vi "Z900_navX_Internal_SendIntegrationControl.vi"(8 "error in (no error)":errorcluster, 9 "Integration Control Register":T7 items=["UNDEFINED"=0, "NAVX_INTEGRATION_CTL_RESET_VEL_X"=1, "NAVX_INTEGRATION_CTL_RESET_VEL_Y"=2, "NAVX_INTEGRATION_CTL_RESET_VEL_Z"=4, "NAVX_INTEGRATION_CTL_RESET_DISP_X"=8, "NAVX_INTEGRATION_CTL_RESET_DISP_Y"=16, "NAVX_INTEGRATION_CTL_RESET_DISP_Z"=32, "NAVX_INTEGRATION_CTL_RESET_YAW"=128], 10 "Interface TypeDefs":T1 {"I2CDevRef"."Device Address" format="%.0x"}, 11 "navX Device":T8={"Interface"={"Protocol"=enum."SERIAL", "Update Rate (4Hz-100Hz)"=4, "navX Open TypeDef"=variant}, "Notify Packet"=refnum, "Loop VI Refnum"=refnum, "Ready to Close Occurrence Refnum"=refnum} {"Interface"."Update Rate (4Hz-100Hz)" min=4 max=60 step=1}) -> (0 "error out":errorcluster, 2 "Interface TypeDefs":T1 {"I2CDevRef"."Device Address" format="%.0x"}, 3 "navX Device":T8={"Interface"={"Protocol"=enum."SERIAL", "Update Rate (4Hz-100Hz)"=4, "navX Open TypeDef"=variant}, "Notify Packet"=refnum, "Loop VI Refnum"=refnum, "Ready to Close Occurrence Refnum"=refnum} {"Interface"."Update Rate (4Hz-100Hz)" min=4 max=60 step=1})   [LabVIEW 2017, in "navX Library v2.lvlib"]
uses:
  navX Library v2.lvlib
  TypeDefs/Z900_navX_DeviceTypeDef.ctl
  TypeDefs/Z900_navX_ProtocolTypeDef.ctl
  TypeDefs/Z900_navX_NotifyPacketTypeDef.ctl
  TypeDefs/Z900_navX_ActionTypeDef.ctl
  TypeDefs/Z900_navX_IntegrationControlRegisters.ctl
  TypeDefs/Z900_navX_InterfaceTypeDef.ctl
  <vilib>/Rock Robotics/WPI/SerialPort/WPI_SerialPortRef.ctl
  <vilib>/Rock Robotics/WPI/I2C/WPI_I2CDevRef.ctl
  <vilib>/Rock Robotics/SystemInterfaces/i2clib/i2c_bus.ctl
  <vilib>/Rock Robotics/WPI/SPI/WPI_SPIDevRef.ctl
  <vilib>/Rock Robotics/SystemInterfaces/spilib/spi_bus.ctl
  TypeDefs/Z900_navX_DeviceRegisters.ctl
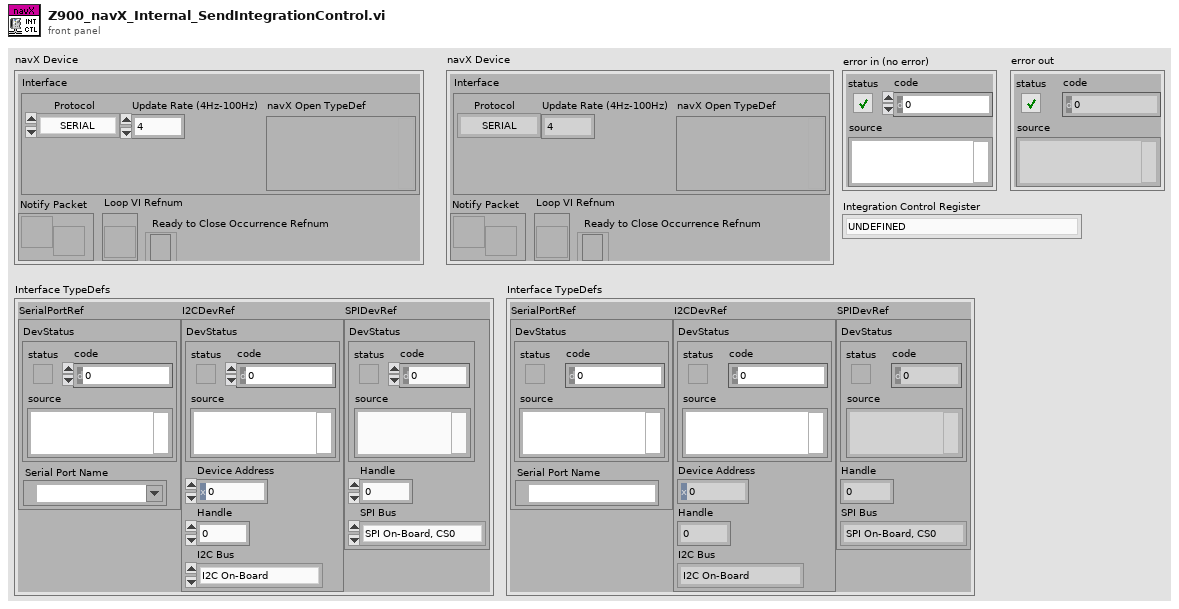
[diagram p1: front panel]
types:
  T1 = typedef "navX Library v2.lvlib/Z900_navX_InterfaceTypeDef.ctl" = cluster{"SerialPortRef":T2, "I2CDevRef":T3, "SPIDevRef":T5}
  T2 = typedef "WPI_SerialPortRef.ctl" = cluster{"DevStatus":errorcluster, "Serial Port Name":refnum<visa-resource-name>}
  T3 = typedef "WPI_I2CDevRef.ctl" = cluster{"DevStatus":errorcluster, "Device Address":u8, "Handle":i32, "I2C Bus":T4}
  T4 = typedef "i2c_bus.ctl" = enum16{"I2C On-Board", "I2C MXP", "Invalid"}
  T5 = typedef "WPI_SPIDevRef.ctl" = cluster{"DevStatus":errorcluster, "Handle":i32, "SPI Bus":T6}
  T6 = typedef "spi_bus.ctl" = enum16{"SPI On-Board, CS0", "SPI On-Board, CS1", "SPI On-Board, CS2", "SPI On-Board, CS3", "SPI MXP", "Invalid"}
  T7 = typedef "navX Library v2.lvlib/Z900_navX_IntegrationControlRegisters.ctl" = u8
  T8 = typedef "navX Library v2.lvlib/Z900_navX_DeviceTypeDef.ctl" = cluster{"Interface":cluster{"Protocol":T9, "Update Rate (4Hz-100Hz)":u8, "navX Open TypeDef":variant}, "Notify Packet":refnum<notifier>, "Loop VI Refnum":refnum<vi>, "Ready to Close Occurrence Refnum":refnum<k4>}
  T9 = typedef "navX Library v2.lvlib/Z900_navX_ProtocolTypeDef.ctl" = enum16{"SERIAL", "I2C", "SPI"}
  T10 = typedef "navX Library v2.lvlib/Z900_navX_DeviceRegisters.ctl" = u8
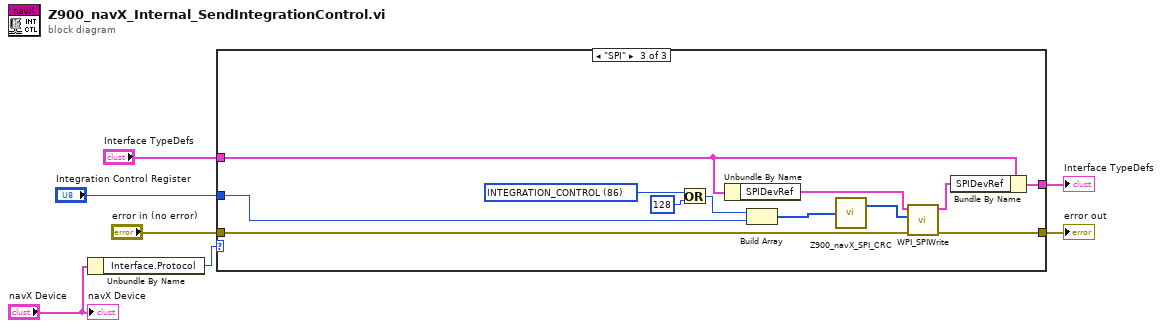
[diagram p0: block diagram]
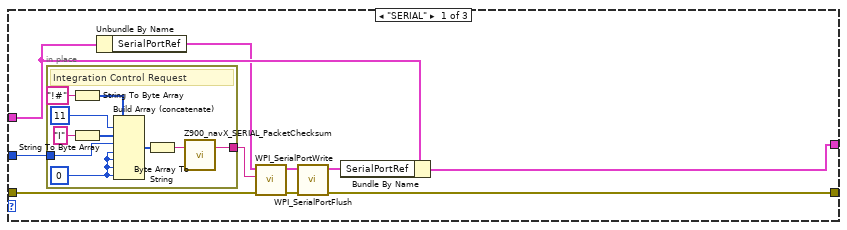
[diagram p2: hidden frame]
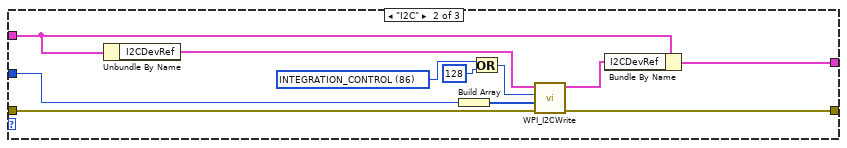
[diagram p3: hidden frame]
diagram:
  n1 = Unbundle By Name("navX Device") -> ("Interface.Protocol"=w6:T9)
  n2 = case shown="\"SPI\"" w6 {
    tunnel: "Interface TypeDefs" -> [w13 w38 w50]
    tunnel: "Integration Control Register" -> [w17 w30 w43]
    tunnel: [w10 w37 w49] -> w3
    tunnel: "error in (no error)" -> [w9 w29 w39]
    tunnel: [w8 w28 w40] -> w1
    frame "SERIAL" {
      n3 = in-place {
        in-place-border: [w20] -> w14
        in-place-border: w17 -> [w18]
        w19 = 0
        # "Integration Control Request"
        n4 = String To Byte Array(string="!#" ("initial string")) -> (unsigned byte array=w25:u8[])
        n5 = String To Byte Array(string="I" ("initial string")) -> (unsigned byte array=w23:u8[])
        n6 = Build Array (concatenate)(w25, 11, w23, w18, w19, w19, w19, w19) -> (w22:i32[])
        n7 = Byte Array To String(unsigned byte array=w22) -> (string=w21:string)
        n8 = call "Z900_navX_SERIAL_PacketChecksum.vi"("Packet"=w21) -> ("Terminated Packet"=w20:string)  [unwired: 1 in, 1 out]
      }
      n9 = Unbundle By Name(w13) -> ("SerialPortRef"=w12:T2)
      n10 = call <vilib>:"WPI_SerialPortWrite.vi"("error in (no error)"=w9, "Buffer"=w14, "SerialPortRef"=w12) -> ("error out"=w16:errorcluster, "SerialPortRef"=w15:T2)  [unwired: 6 in, 1 out]
      n11 = call <vilib>:"WPI_SerialPortFlush.vi"("error in (no error)"=w16, "SerialPortRef"=w15) -> ("error out"=w8:errorcluster, "SerialPortRef"=w11:T2)  [unwired: 8 in]
      n12 = Bundle By Name(cluster=w13, "SerialPortRef"=w11) -> (w10:T1)
    }
    frame "I2C" {
      w34 = T10 86 items=["WHOAMI"=0, "HW_REV"=1, "FW_VER_MAJOR"=2, "FW_VER_MINOR"=3, "UPDATE_RATE_HZ"=4, "ACCEL_FSR_G"=5, "GYRO_FSR_DPS"=6, "OP_STATUS"=8, "CAL_STATUS"=9, "SELFTEST_STATUS"=10, "CAPABILITY_FLAGS_L"=11, "CAPABILITY_FLAGS_H"=12, "SENSOR_STATUS"=16, "TIMESTAMP"=18, "YAW"=22, "ROLL"=24, "PITCH"=26, "HEADING"=28, "FUSED_HEADING"=30, "ALTITUDE_I"=32, "ALTITUDE_D"=34, "LINERA_ACC_X"=36, "LINERA_ACC_Y"=38, "LINERA_ACC_Z"=40, "QUAT_W"=42, "QUAT_X"=44, "QUAT_Y"=46, "QUAT_Z"=48, "MPU_TEMP_C"=50, "GYRO_X"=52, "GYRO_Y"=54, "GYRO_Z"=56, "ACC_X"=58, "ACC_Y"=60, "ACC_Z"=62, "MAG_X"=64, "MAG_Y"=66, "MAG_Z"=68, "PRESSURE_I"=70, "PRESSURE_D"=72, "PRESSURE_TEMP"=74, "YAW_OFFSET"=76, "QUAT_OFFSET_W"=78, "QUAT_OFFSET_X"=80, "QUAT_OFFSET_Y"=82, "QUAT_OFFSET_Z"=84, "INTEGRATION_CONTROL"=86, "VELOCITY_X"=88, "VELOCITY_Y"=92, "VELOCITY_Z"=96, "DISPLACMENT_X"=100, "DISPLACMENT_Y"=104, "DISPLACEMENT_Z"=108] ("Device Register")
      n13 = Unbundle By Name(w38) -> ("I2CDevRef"=w36:T3)
      n14 = Build Array(w30) -> (w32:T7[])
      n15 = Or(x=w34, y=u8 128) -> (x .or. y?=w33:T10)
      n16 = call <vilib>:"WPI_I2CWrite.vi"("error in (no error)"=w29, "I2CDataToSend"=w32, "I2CRegister"=w33, "I2CDevRef"=w36) -> ("error out"=w28:errorcluster, "I2CDevRef"=w35:T3)  [unwired: 6 in]
      n17 = Bundle By Name(cluster=w38, "I2CDevRef"=w35) -> (w37:T1)
    }
    frame "SPI" {
      w44 = T10 86 items=["WHOAMI"=0, "HW_REV"=1, "FW_VER_MAJOR"=2, "FW_VER_MINOR"=3, "UPDATE_RATE_HZ"=4, "ACCEL_FSR_G"=5, "GYRO_FSR_DPS"=6, "OP_STATUS"=8, "CAL_STATUS"=9, "SELFTEST_STATUS"=10, "CAPABILITY_FLAGS_L"=11, "CAPABILITY_FLAGS_H"=12, "SENSOR_STATUS"=16, "TIMESTAMP"=18, "YAW"=22, "ROLL"=24, "PITCH"=26, "HEADING"=28, "FUSED_HEADING"=30, "ALTITUDE_I"=32, "ALTITUDE_D"=34, "LINERA_ACC_X"=36, "LINERA_ACC_Y"=38, "LINERA_ACC_Z"=40, "QUAT_W"=42, "QUAT_X"=44, "QUAT_Y"=46, "QUAT_Z"=48, "MPU_TEMP_C"=50, "GYRO_X"=52, "GYRO_Y"=54, "GYRO_Z"=56, "ACC_X"=58, "ACC_Y"=60, "ACC_Z"=62, "MAG_X"=64, "MAG_Y"=66, "MAG_Z"=68, "PRESSURE_I"=70, "PRESSURE_D"=72, "PRESSURE_TEMP"=74, "YAW_OFFSET"=76, "QUAT_OFFSET_W"=78, "QUAT_OFFSET_X"=80, "QUAT_OFFSET_Y"=82, "QUAT_OFFSET_Z"=84, "INTEGRATION_CONTROL"=86, "VELOCITY_X"=88, "VELOCITY_Y"=92, "VELOCITY_Z"=96, "DISPLACMENT_X"=100, "DISPLACMENT_Y"=104, "DISPLACEMENT_Z"=108] ("Device Register")
      n18 = Or(x=w44, y=u8 128) -> (x .or. y?=w46:T10)
      n19 = Unbundle By Name(w50) -> ("SPIDevRef"=w42:T5)
      n20 = Build Array(w46, w43) -> (w47:T7[])
      n21 = call "Z900_navX_SPI_CRC.vi"("Message"=w47) -> ("Message with CRC"=w48:u8[])  [unwired: 1 out]
      n22 = call <vilib>:"WPI_SPIWrite.vi"("error in (no error)"=w39, "Data To Send"=w48, "SPIDevRef"=w42) -> ("error out"=w40:errorcluster, "SPIDevRef"=w41:T5)  [unwired: 6 in, 1 out]
      n23 = Bundle By Name(cluster=w50, "SPIDevRef"=w41) -> (w49:T1)
    }
  }
  "error out" <- w1
  "Interface TypeDefs" <- w3
  "navX Device" <- "navX Device"
